vi "MSEditor_MethodFGV.vi"(1 "Mthd in":T1, 3 "error in (no error)":errorcluster, 4 "Function":enum16{"Write", "Read"}(ring)=enum."Read") -> (8 "Mthd out":T1, 10 "error out":errorcluster)   [LabVIEW 2018]
uses:
  PublicSubVI/Class/SigInfo/SigInfo.lvclass
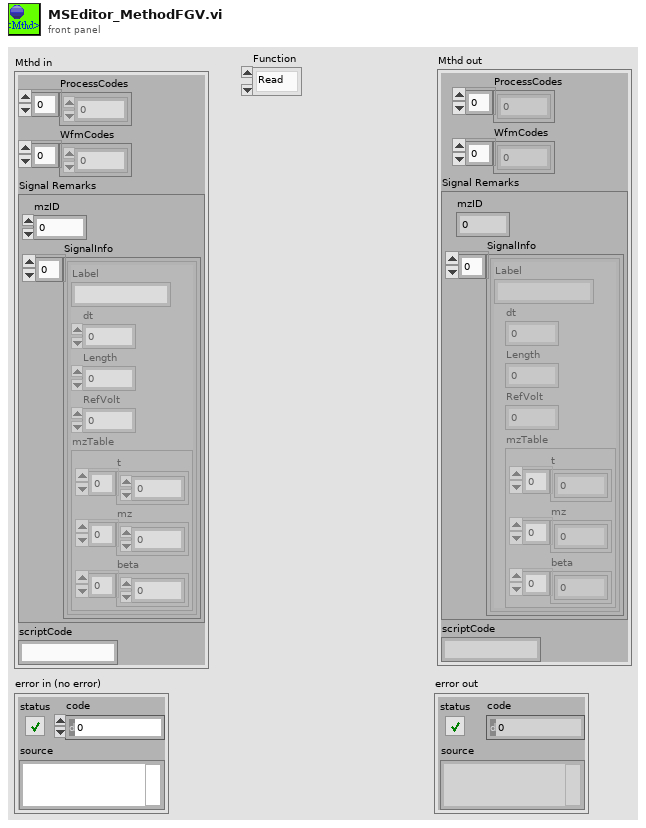
[diagram p1: front panel]
types:
  T1 = cluster{"ProcessCodes":u64[], "WfmCodes":u64[], "Signal Remarks":cluster{"mzID":u64, "SignalInfo":cluster{"Label":string, "dt":dbl, "Length":u32, "RefVolt":dbl, "mzTable":cluster{"t":dbl[], "mz":dbl[], "beta":dbl[]}}[]}, "scriptCode":string}
  T2 = enum16{"New mzList", "Set SigInfo", "Get SigInfo", "Append", "End"}
  T3 = cluster{"mzID":u64, "SignalInfo":cluster{"Label":string, "dt":dbl, "Length":u32, "RefVolt":dbl, "mzTable":cluster{"t":dbl[], "mz":dbl[], "beta":dbl[]}}[]}
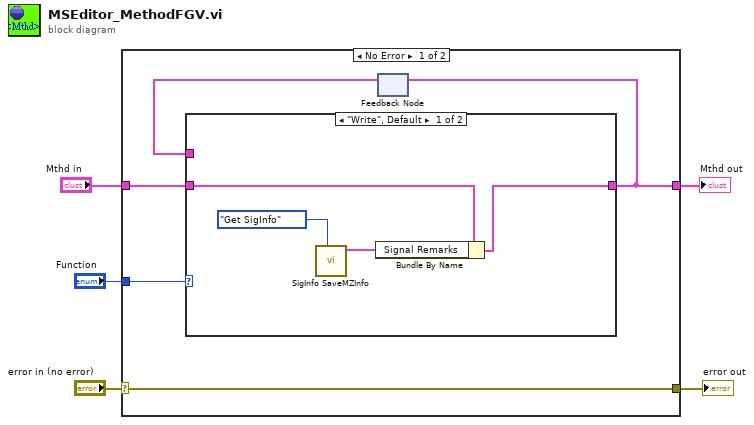
[diagram p0: block diagram]
diagram:
  n1 = case shown="No Error" "error in (no error)" {
    selector: "error in (no error)" -> [w6 w16]
    tunnel: "Function" -> [w10 _]
    tunnel: "Mthd in" -> [w9 w17]
    tunnel: [w8 w17] -> w1
    tunnel: [w6 w16] -> w3
    frame No Error {
      n2 = feedback #1() -> (w7:T1)  [unwired: 1 in]
      n3 = case shown="\"Write\", Default" w10 {
        tunnel: w9 -> [w13 _]
        tunnel: [w11 w15] -> w8
        tunnel: w7 -> [_ w15]
        frame "Write", Default {
          n4 = call "SigInfo SaveMZInfo.vi"("Function"=T2."Get SigInfo") -> ("Signal Remarks output"=w12:T3)  [unwired: 8 in, 2 out]
          n5 = Bundle By Name(cluster=w13, "Signal Remarks"=w12) -> (w11:T1)
        }
        frame "Read" {
        }
      }
      n6 = feedback-in #1(w8) -> ()
    }
    frame Error {
    }
  }
  "error out" <- w3
  "Mthd out" <- w1
